vi "Read Values.vi"(8 "error in (no error)":errorcluster, 11 "Log Write Message in":refnum<class "Log Write Message.lvclass">) -> (0 "error out":errorcluster, 2 "Values":dbl[](array[numeric]), 3 "Log Write Message out":refnum<class "Log Write Message.lvclass">)   [LabVIEW 2017, in "Messaging.lvlib" / "Log Write Message.lvclass"]
uses:
  Log Write Message.lvclass
  Log Write Message.lvclass/Log Write Message.ctl
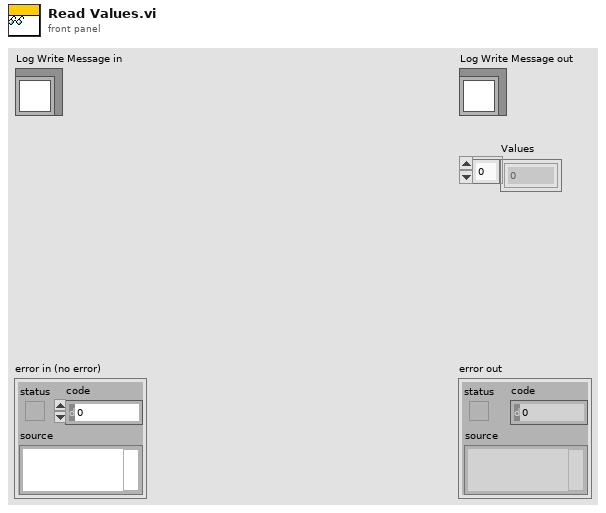
[diagram p1: front panel]
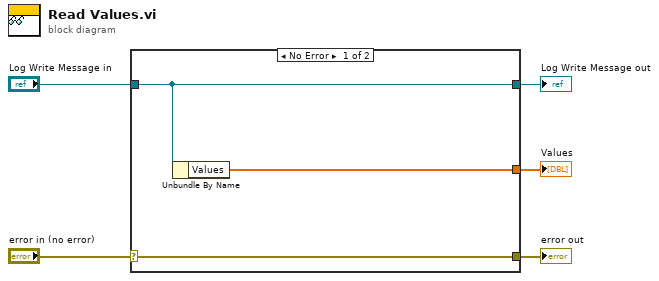
[diagram p0: block diagram]
diagram:
  n1 = case shown="No Error" "error in (no error)" {
    selector: "error in (no error)" -> [w8 w9]
    tunnel: [w8 w9] -> w4
    tunnel: [w7 w10] -> w2
    tunnel: "Log Write Message in" -> [w7 w10]
    tunnel: [w6 _] -> w1
    frame No Error {
      n2 = Unbundle By Name(w7) -> ("Values"=w6:dbl[])
    }
    frame Error {
    }
  }
  "error out" <- w4
  "Log Write Message out" <- w2
  "Values" <- w1
